vi "Query Assets with Filter.vi"(8 "Error in":errorcluster, 10 "Filter string":string, 11 "NI Skyline Configuration HTTP in":refnum<class "NI Skyline Configuration HTTP.lvclass">) -> (0 "Error out":errorcluster, 2 "Assets":T1 {"assets"."externalCalibration"."nextRecommendedDate" format="%<%x>T"; "assets"."externalCalibration"."date" format="%<%x>T"}, 3 "NI Skyline Configuration HTTP out":refnum<class "NI Skyline Configuration HTTP.lvclass">)   [LabVIEW 2020]
uses:
  <vilib>/Skyline/Configuration/Configuration HTTP_class/NI Skyline Configuration HTTP.lvclass
  Assets.ctl
  Asset.ctl
  externalCalibration.ctl
  <vilib>/Skyline/Configuration/Configuration HTTP_class/NI Skyline Configuration HTTP.lvclass/NI Skyline Configuration HTTP.ctl
  <vilib>/Skyline/Configuration/Configuration HTTP_class/Read Server URL.vi
  <vilib>/httpClient/POSTBuffer.vi
  <vilib>/regexp/Match Regular Expression.xnode
  <vilib>/httpClient/LabVIEWHTTPClient.lvlib
  <vilib>/addons/_JKI.lib/Serialization/JSON/JKI JSON Serialization.lvlib
panel:
  out "body":string
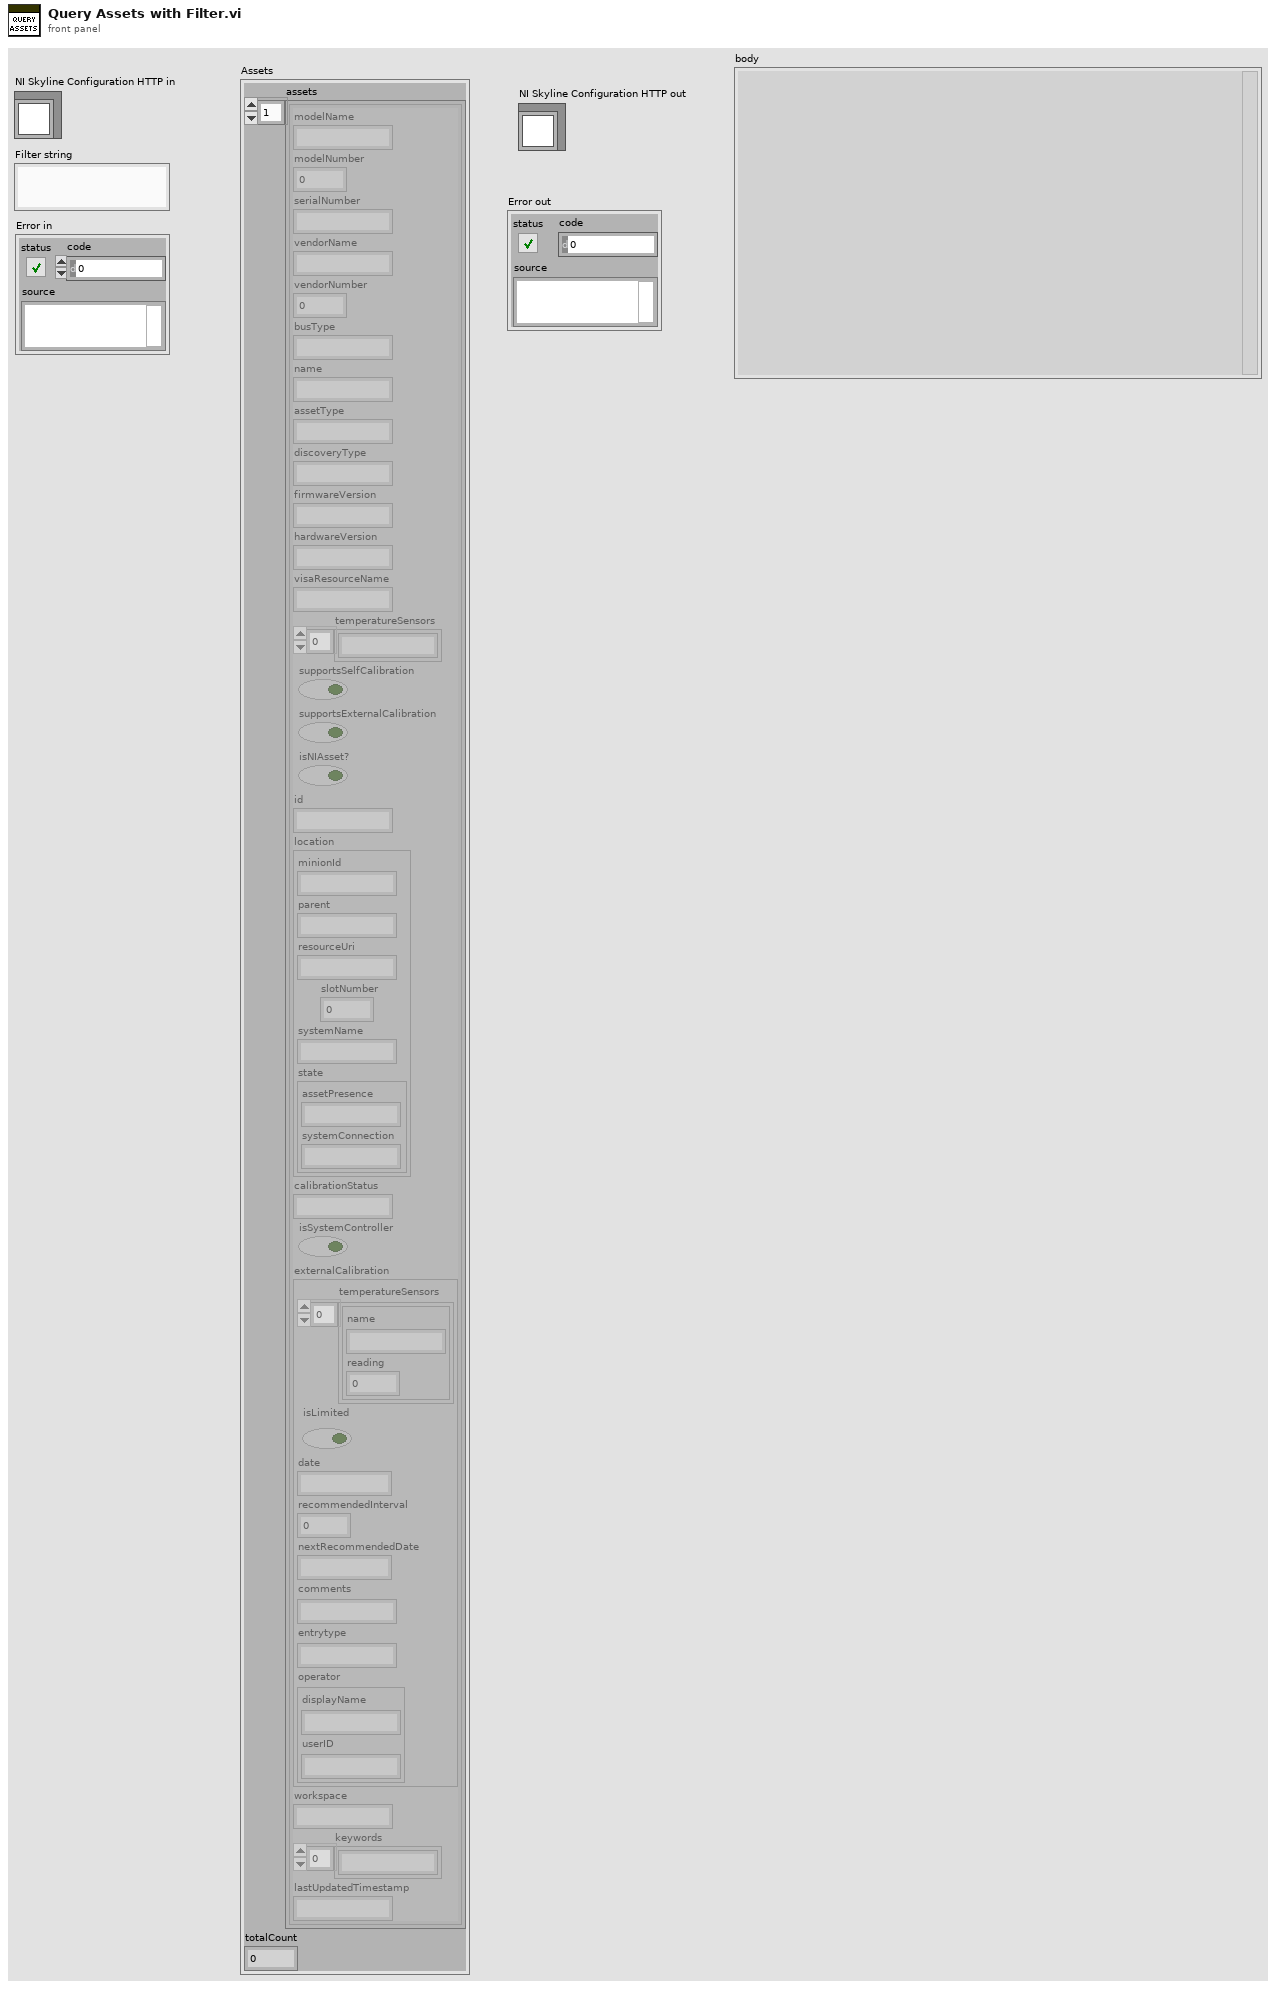
[diagram p1: front panel]
types:
  T1 = typedef "Assets.ctl" = cluster{"assets":T2[], "totalCount":u64}
  T2 = typedef "Asset.ctl" = cluster{"modelName":string, "modelNumber":u64, "serialNumber":string, "vendorName":string, "vendorNumber":u64, "busType":string, "name":string, "assetType":string, "discoveryType":string, "firmwareVersion":string, "hardwareVersion":string, "visaResourceName":string, "temperatureSensors":string[], "supportsSelfCalibration":bool, "supportsExternalCalibration":bool, "isNIAsset?":bool, "id":string, "location":cluster{"minionId":string, "parent":string, "resourceUri":string, "slotNumber":u64, "systemName":string, "state":cluster{"assetPresence":string, "systemConnection":string}}, "calibrationStatus":string, "isSystemController":bool, "externalCalibration":T3, "workspace":string, "keywords":string[], "lastUpdatedTimestamp":string}
  T3 = typedef "externalCalibration.ctl" = cluster{"temperatureSensors":cluster{"name":string, "reading":dbl}[], "isLimited":bool, "date":timestamp, "recommendedInterval":i32, "nextRecommendedDate":timestamp, "comments":string, "entrytype":string, "operator":cluster{"displayName":string, "userID":string}}
  T4 = typedef "LabVIEWHTTPClient.lvlib/ClientHandle.ctl" = refnum<k1>
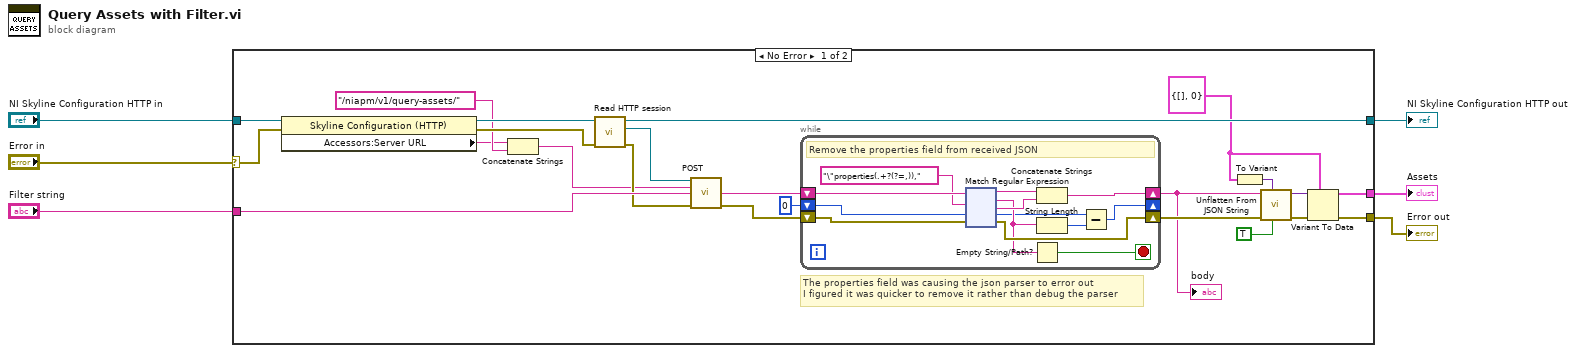
[diagram p0: block diagram]
diagram:
  n1 = case shown="No Error" "Error in" {
    selector: "Error in" -> [w8 w158]
    tunnel: [w29 w158] -> w6
    tunnel: [w28 _] -> w1
    tunnel: "Filter string" -> [w18 _]
    tunnel: "NI Skyline Configuration HTTP in" -> [w10 w157]
    tunnel: [w9 w157] -> w3
    frame No Error {
      w7 = T1 {"assets"=[], "totalCount"=0} ("Assets")
      # "The properties field was causing the json parser to error out\nI figured it was quicker to remove it rather than debug the parser"
      n2 = property class="Skyline Configuration (HTTP)"(reference=w10, error in=w8) -> (reference out=w13:refnum<class "NI Skyline Configuration HTTP.lvclass">, error out=w14:errorcluster, "Accessors:Server URL"=w11:string)
      n3 = Concatenate Strings(w11, "/niapm/v1/query-assets/" ("initial string")) -> (w16:string)
      n4 = call <vilib>:"Read HTTP session.vi"("error in (no error)"=w14, "HTTP configuration in"=w13) -> ("error out"=w17:errorcluster, "http session"=w15:T4, "HTTP configuration out"=w9:refnum<class "NI Skyline Configuration HTTP.lvclass">)  [unwired: 7 in]
      n5 = call-poly <vilib>:"POST.vi"("client handle"=w15, "url"=w16, "buffer"=w18, "error in (no error)"=w17) -> ("body"=w19:string, "error out"=w23:errorcluster)  [unwired: 8 in, 2 out]
      n6 = while {
        shift-right: [w40] -> w20
        shift-left: w19 -> [w39]
        shift-right: [w37] -> w21
        shift-left: w23 -> [w36]
        shift-right: [w32] -> _
        shift-left: 0 -> [w31]
        stop <- w30 stop-if-true
        # "Remove the properties field from received JSON"
        n7 = xnode "Match Regular Expression"("input string"=w39, "regular expression"="\"properties(.+?(?=,)),", "offset (0)"=w31, "error in"=w36) -> ("before match"=w41:string, "whole match"=w35:string, "after match"=w42:string, "offset past match"=w34:i32, "error out"=w37:errorcluster)  [unwired: 2 in]
        n8 = Empty String/Path?(string/path=w35) -> (empty?=w30:bool)
        n9 = Concatenate Strings(w41, w42) -> (w40:string)
        n10 = String Length(string=w35) -> (length=w33:i32)
        n11 = Subtract(x=w34, y=w33) -> (x-y=w32:i32)
      }
      "body" <- w20
      n12 = To Variant(anything=w7) -> (Variant=w25:variant)
      n13 = call <vilib>:"Unflatten From JSON String.vi"("Nulls as Defaults (F)"=TRUE, "Type and Defaults"=w25, "error in (no error)"=w21, "JSON String"=w20) -> ("error out"=w27:errorcluster, "Variant"=w26:variant)  [unwired: 6 in]
      n14 = Variant To Data(error in=w27, type=w7, Variant=w26) -> (data=w28:T1, error out=w29:errorcluster)
    }
    frame Error {
    }
  }
  "Assets" <- w1
  "Error out" <- w6
  "NI Skyline Configuration HTTP out" <- w3
